vi "002 Data Forwarding Module.vi"(11 "Queue Ref In":T1={"UI"=refnum, "Message"=refnum, "Data"=refnum, "Caller"=refnum, "Name"="000 Common", "Data Path"=path "", "Class Path"=path "", "SubPanel"=refnum, "Project Name"="", "MNT"="", "Title"="", "Data Source"=refnum, "Queue List"={}, "VI"=refnum, "UE"=refnum}) -> ()   [LabVIEW 2020]
doc: "002 Data Forwarding Module.vi"
uses:
  Alin/QMH/000 Module Data Type.ctl
  Alin/QMH/Queue Message.ctl
  <vilib>/Utility/file.llb/Read Delimited Spreadsheet (string).vi
panel:
  in  "Forwarding Interval":u32=1000 caption="转发间隔(ms)" min=500 max=100000 step=1
  out "Name":string
  in  "Forward List":T2(array[cluster])
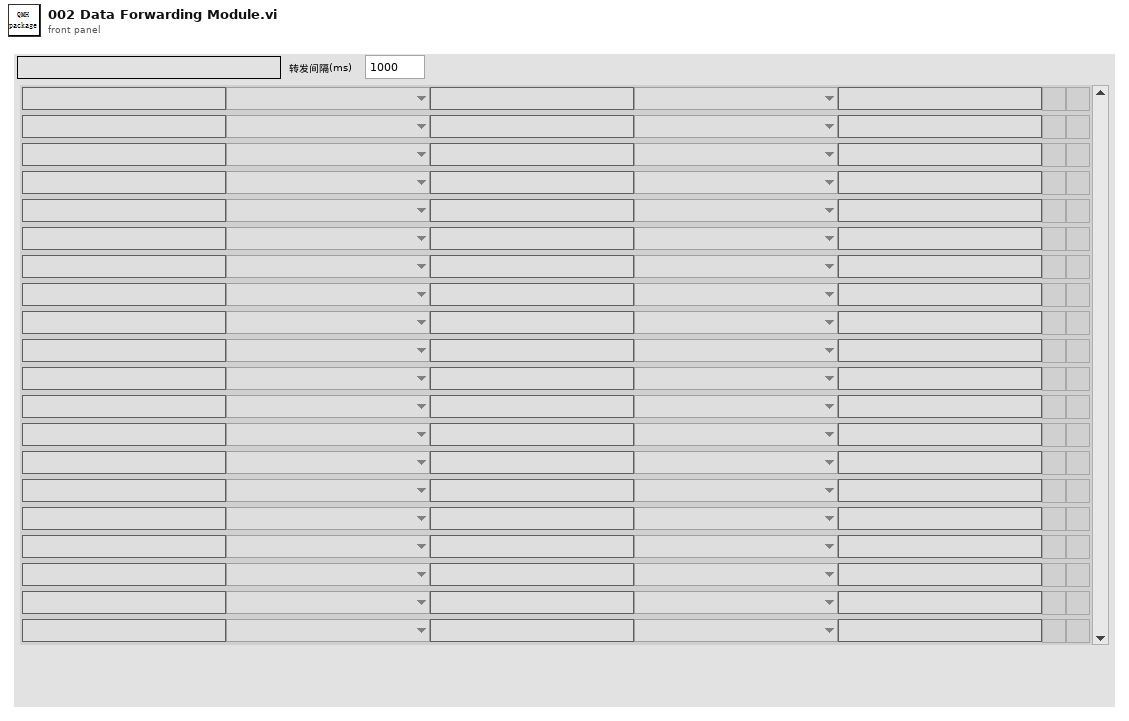
[diagram p1: front panel]
types:
  T1 = typedef "000 Module Data Type.ctl" = cluster{"UI":refnum<queue>, "Message":refnum<queue>, "Data":refnum<queue>, "Caller":refnum<queue>, "Name":string, "Data Path":path, "Class Path":path, "SubPanel":refnum<vi>, "Project Name":string, "MNT":string, "Title":string, "Data Source":refnum<queue>, "Queue List":map{string, refnum<queue>}, "VI":refnum<vi>, "UE":refnum<user-event>}
  T2 = cluster{"Name":string, "Sender":u16, "Send ID":string, "Receiver":u16, "Receive ID":string, "Edit":bool, "Delete":bool}[]
  T3 = cluster{"Queue":T1, "Delay":cluster{"Count Time(ms)":u32, "Delay Time(ms)":u32, "Next":string}, "Panel Name":string[], "Interval":u32, "Forward":map{string, cluster{"Name":string, "Sender":string, "SendID":string, "Receiver":string, "ReceiverID":string}}, "Group":map{string, map{string, cluster{"Name":string, "Sender":string, "SendID":string, "Receiver":string, "ReceiverID":string}}}, "Type":map{string, string}}
  T4 = map{string, cluster{"Name":string, "Sender":string, "SendID":string, "Receiver":string, "ReceiverID":string}}
  T5 = cluster{"all rows[0]":string, "all rows[1]":string, "all rows[2]":string, "all rows[3]":string, "all rows[4]":string}
  T6 = cluster{"Name":string, "Sender":string, "SendID":string, "Receiver":string, "ReceiverID":string}
  T7 = map{string, map{string, cluster{"Name":string, "Sender":string, "SendID":string, "Receiver":string, "ReceiverID":string}}}
  T8 = typedef "SDQ Data Type.ctl" = cluster{"CAN Length":string, "CAN Name":string, "CAN ID":string, "CAN Type":string, "Test Item":string, "Byte Order":string, "Instruction":string, "Control Type":string, "Group":string, "Offset":dbl, "Coefficient":dbl, "Write Enable":bool, "Lable Type":string, "Key?":string, "Set Value":string, "Upper":dbl, "Lower":dbl, "Unit":string, "Formula":string, "Test Item Type":string, "Length":i32, "Address":string, "Name":string, "Identifier":string, "Data Type":string, "Enumerate?":string, "Enumerate List":string, "Data":string, "Source":string}
  T9 = cluster{"Queue":T1, "Panel Name":string[], "Sender":refnum<vi>, "Receiver":refnum<vi>}
  T10 = typedef "eventvkey.ctl" = enum16{"ASCII", "Enter", "Return", "Shift", "Ctrl", "Alt", "Cmd", "Opt", "Caps", "NumLock", "Clear", "Break", "Up", "Down", "Left", "Right", "Insert", "Delete", "Home", "End", "PageUp", "PageDown", "Escape", "Help", "Pause", "ScrollLock", "F1", "F2", "F3", "F4", "F5", "F6", "F7", "F8", "F9", "F10", "F11", "F12", "F13", "F14", "F15", "F16", "F17", "F18", "F19", "F20", "F21", "F22", "F23", "F24", "Play", "VolumeUp", "VolumeDown", "Mute", "Two Byte Char"}
  T11 = cluster{"Shift":bool, "Ctrl":bool, "Alt":bool, "Cmd":bool, "Opt":bool}
  T12 = typedef "LVPoint32TypeDef.ctl" = cluster{"Horizontal":i32, "Vertical":i32}
  T13 = typedef "LVPositionTypeDef.ctl" = cluster{"Left":i32, "Top":i32}
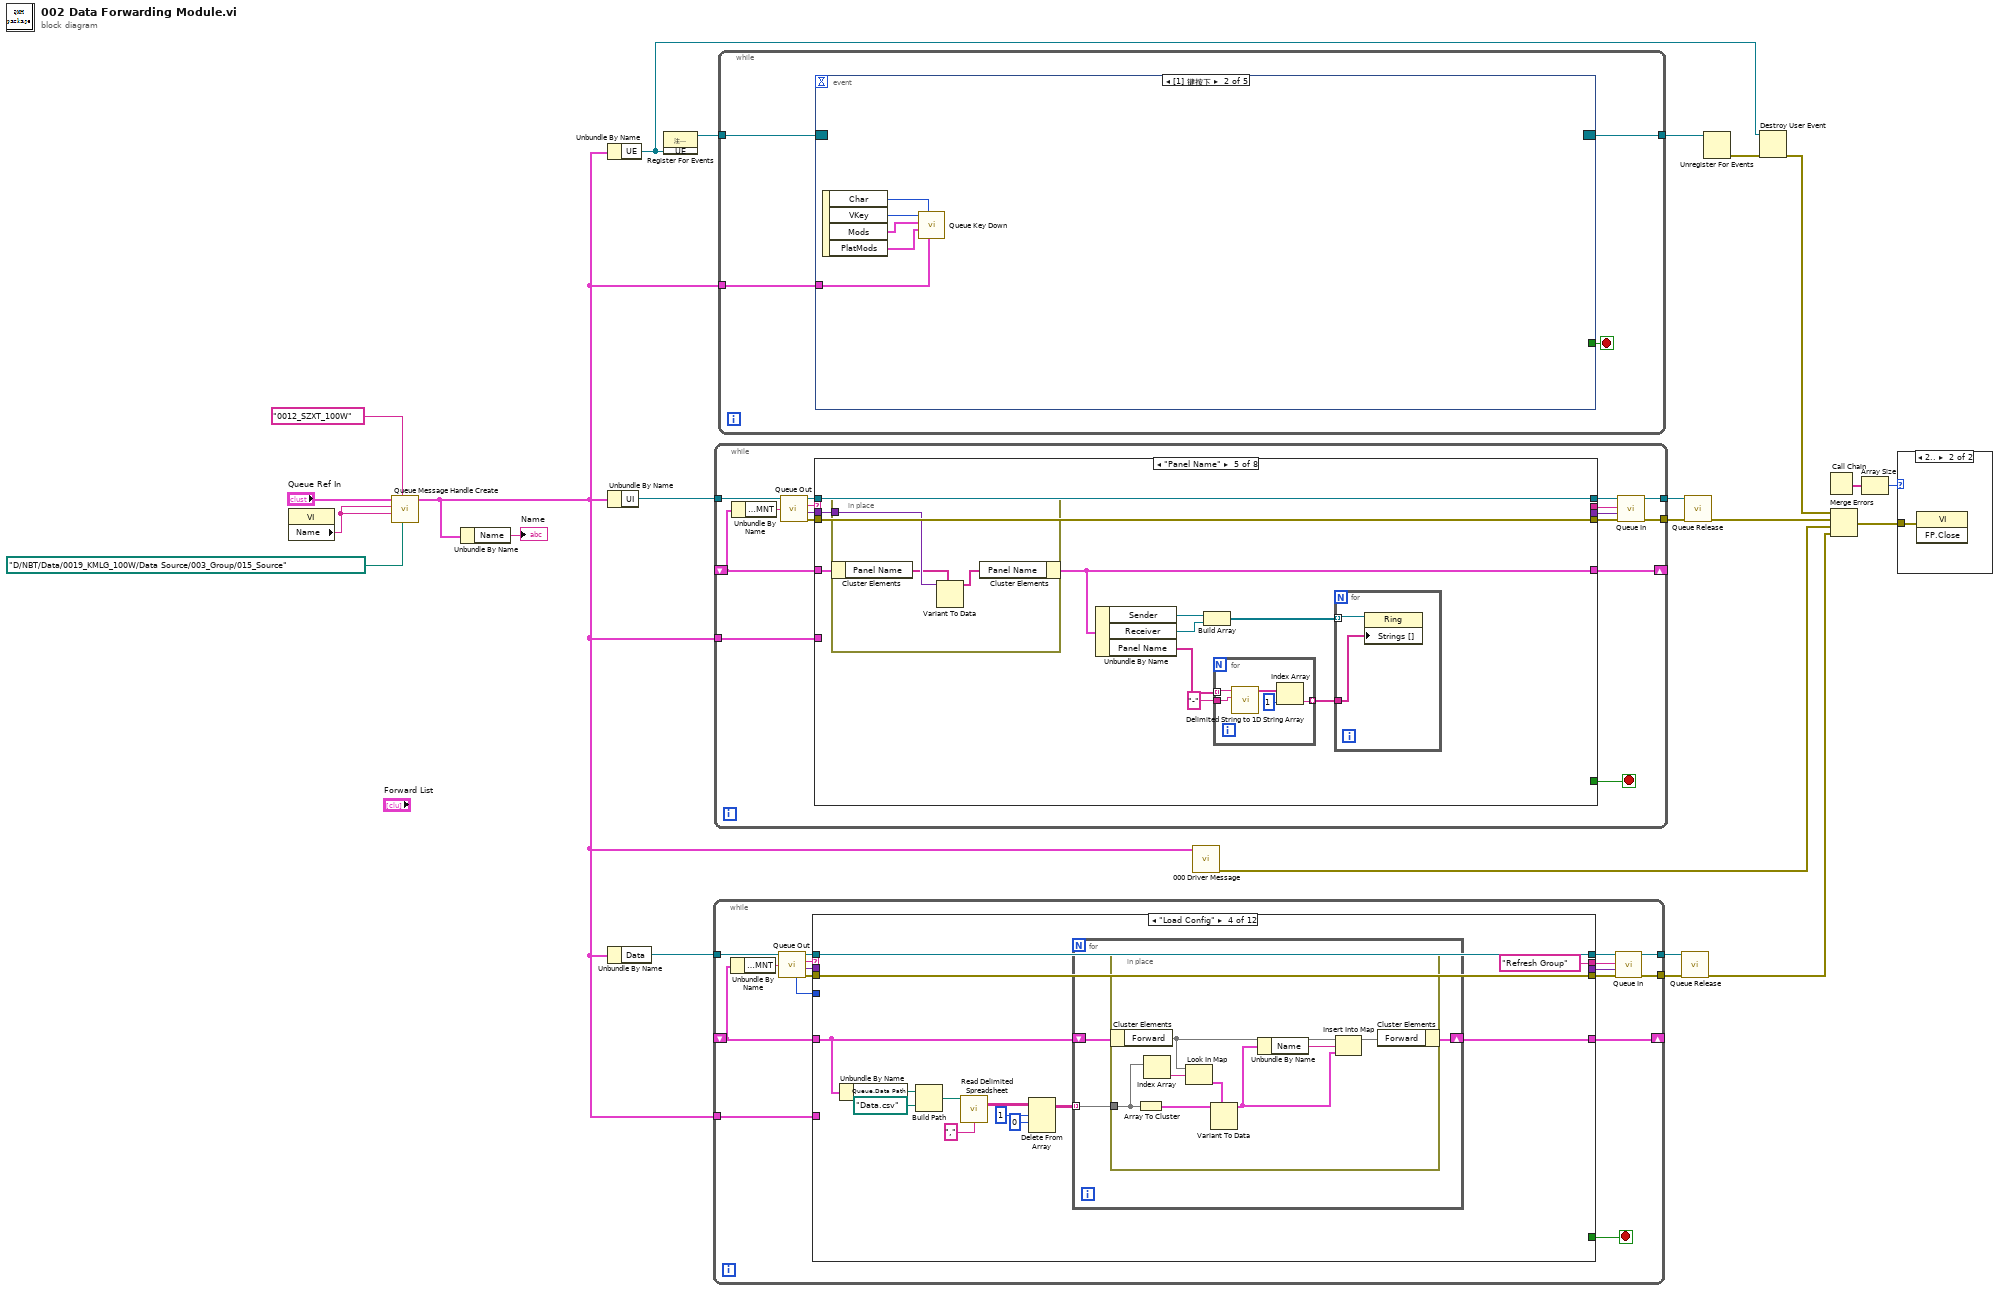
[diagram p0: block diagram]
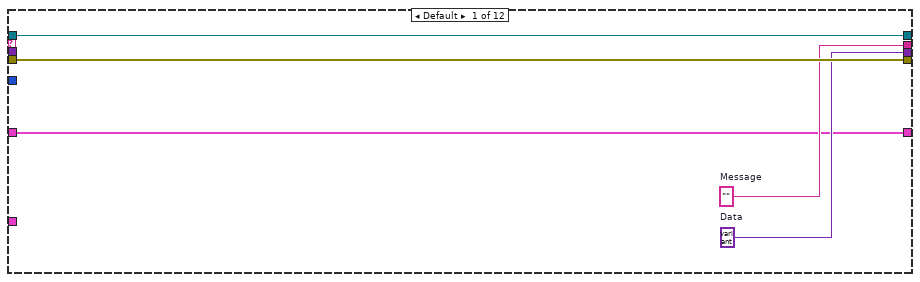
[diagram p2: hidden frame]
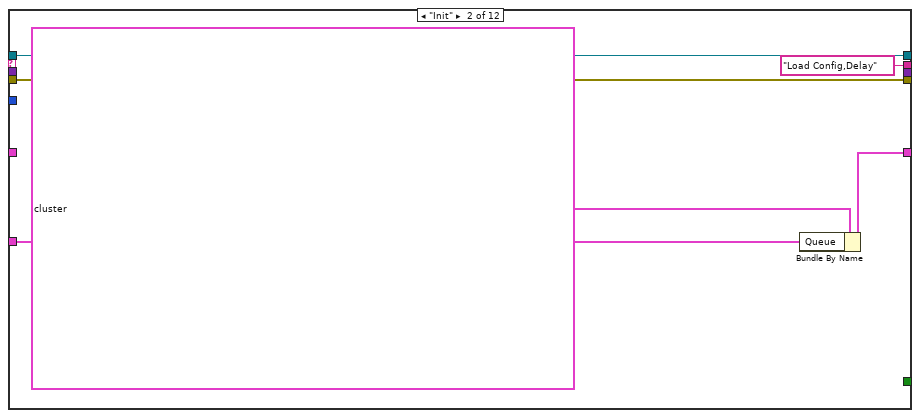
[diagram p3: hidden frame]
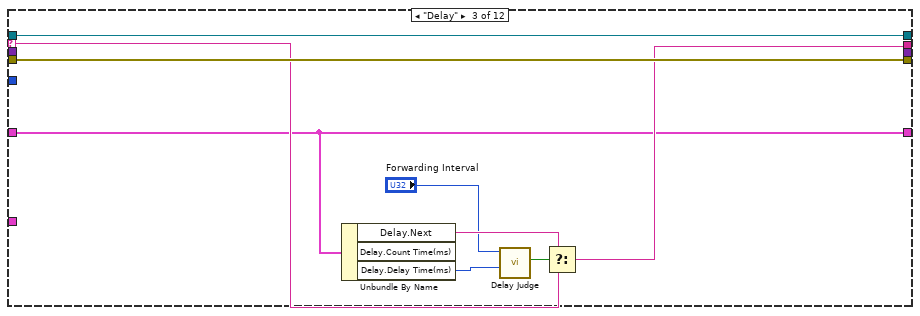
[diagram p4: hidden frame]
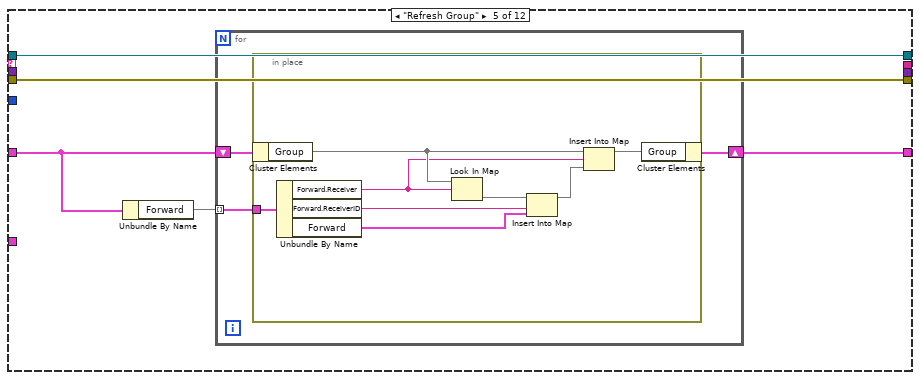
[diagram p5: hidden frame]
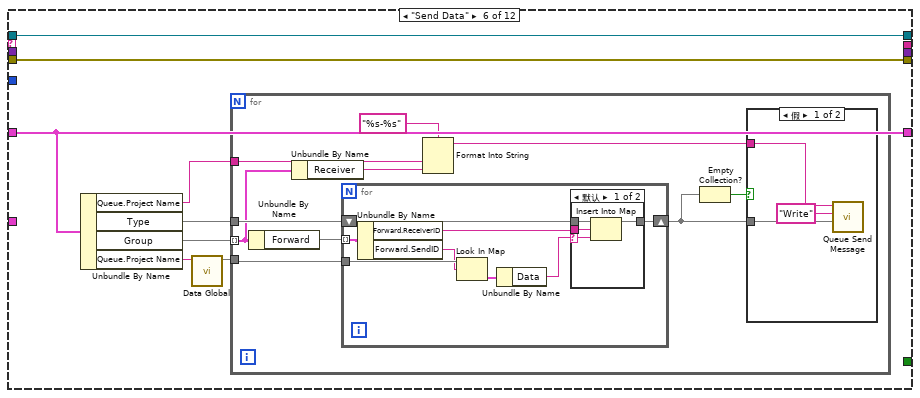
[diagram p6: hidden frame]
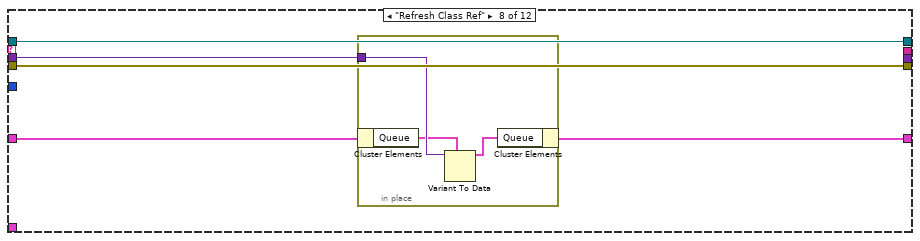
[diagram p10: hidden frame]
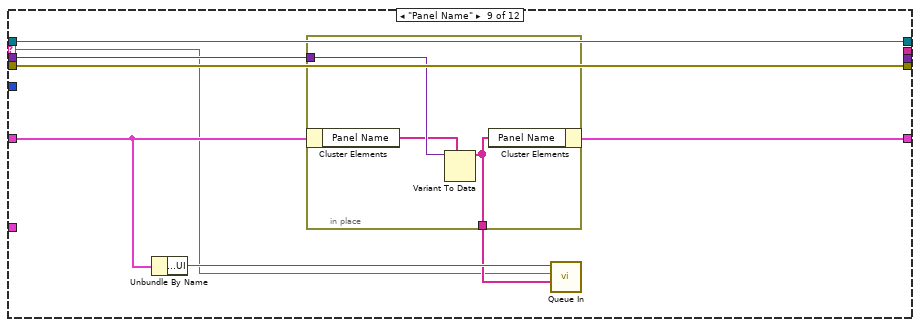
[diagram p11: hidden frame]
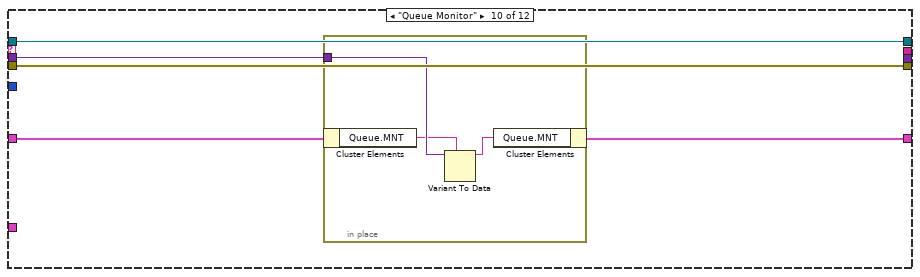
[diagram p12: hidden frame]
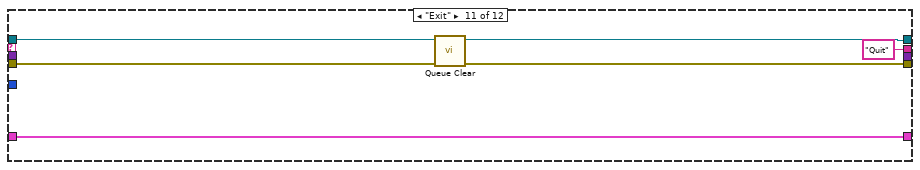
[diagram p13: hidden frame]
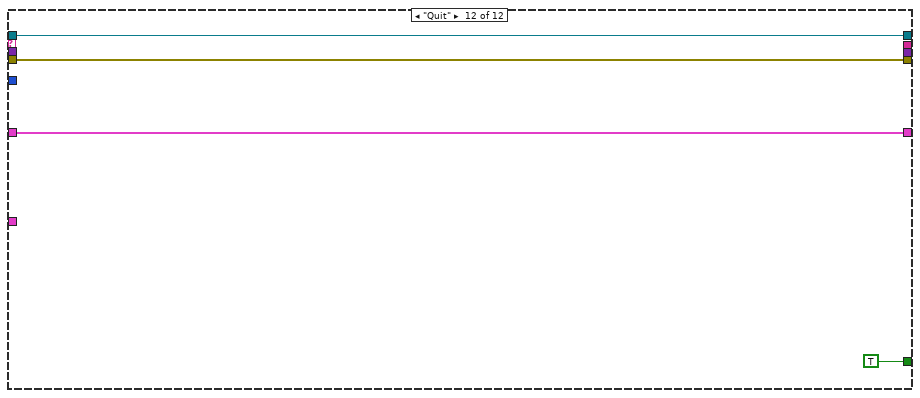
[diagram p14: hidden frame]
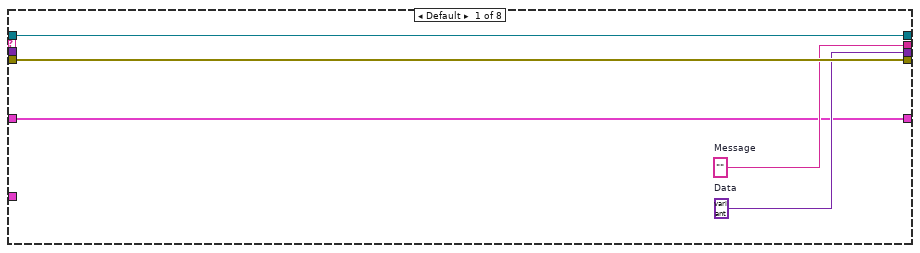
[diagram p16: hidden frame]
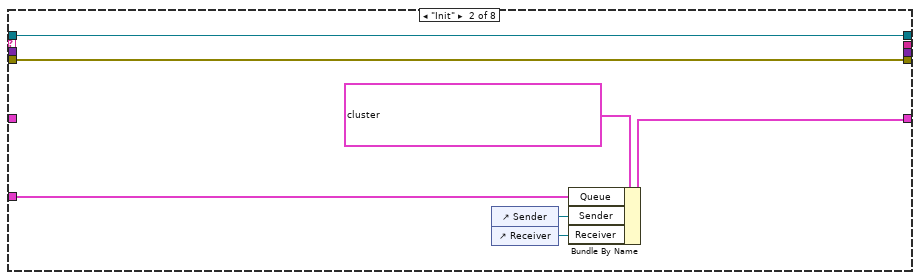
[diagram p17: hidden frame]
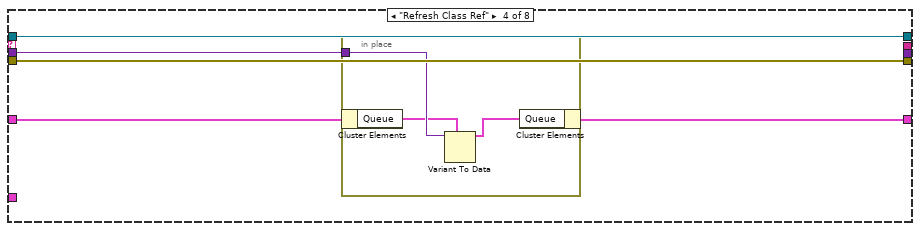
[diagram p19: hidden frame]
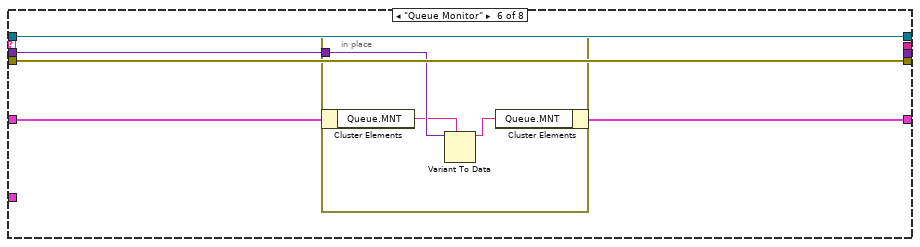
[diagram p20: hidden frame]
diagram:
  n1 = property class="VI"() -> ("Name"=w1:string)  [unwired: 2 in, 2 out]
  n2 = call "Queue Message Handle Create.vi"("Data Path"=path "D:/NBT/Data/0019_KMLG_100W/Data Source/003_Group/015_Source", "Project Name"="0012_SZXT_100W", "Name"=w1, "Title"=w1, "Queue Ref In"="Queue Ref In") -> ("Queue Ref Out"=w4:T1)  [unwired: 5 in, 1 out]
  n3 = Unbundle By Name(w4) -> ("Name"=→"Name":string)
  n4 = Unbundle By Name(w4) -> ("UE"=w7:refnum<user-event>)
  n5 = Unbundle By Name(w4) -> ("UI"=w18:refnum<queue>)
  n6 = Unbundle By Name(w4) -> ("Data"=w10:refnum<queue>)
  n7 = register-events(w7) -> (reference out=w23:refnum<event-registration>)  [unwired: 2 in, 1 out]
  n8 = while {
    tunnel: w10 -> [w36]
    tunnel: [w33] -> w12
    tunnel: [w32] -> w11
    shift-right: [w28] -> _
    shift-left: _ -> [w25]
    tunnel: w4 -> [w24]
    stop <- w40 stop-if-true
    n9 = Unbundle By Name(w25) -> ("Queue.MNT"=w26:string)
    n10 = call "Queue Out.vi"("Monitor"=w26, "Queue In"=w36) -> ("error out"=w39:errorcluster, "Data"=w37:variant, "Message"=w38:string, "Queue Out"=w35:refnum<queue>, "Queue NUmber"=w27:i32)  [unwired: 5 in]
    n11 = case shown="\"Load Config\"" w38 {
      selector: w38 -> [_ _ w54 _ _ _ _ _ w146 _ _ _]
      tunnel: w35 -> [w45 w51 w60 w73 w89 w108 w137 w142 w153 w161 w169 w173]
      tunnel: w39 -> [w44 w50 w59 w72 w88 w107 w136 w141 w152 w160 w167 w174]
      tunnel: [w45 w51 w60 w73 w89 w108 w137 w142 w153 w161 w168 w173] -> w34
      tunnel: [w44 w50 w59 w72 w88 w107 w136 w141 w152 w160 w166 w174] -> w31
      tunnel: [w43 "Load Config,Delay" ("Next") w55 "Refresh Group" ("Next") _ _ _ _ _ _ "Quit" _] -> w30
      tunnel: [_ _ _ _ _ _ _ _ _ _ _ TRUE] -> w40
      tunnel: [w42 _ _ _ _ _ _ _ _ _ _ _] -> w29
      tunnel: w37 -> [_ _ _ _ _ _ _ w138 w150 w157 _ _]
      tunnel: [w41 w47 w53 w63 w85 w106 w135 w139 w151 w158 w165 w171] -> w28
      tunnel: w25 -> [w41 _ w53 w64 w86 w106 w135 w140 w149 w159 w165 w171]
      tunnel: w27 -> [_ _ _ _ _ _ _ _ _ _ _ _]
      tunnel: w24 -> [_ w46 _ _ _ _ _ _ _ _ _ _]
      frame Default {
        w42 = variant  # Data
        w43 = ""  # Message
      }
      frame "Init" {
        n12 = Bundle By Name(cluster=T3 {"Queue"={"UI"=refnum, "Message"=refnum, "Data"=refnum, "Caller"=refnum, "Name"="000 Common", "Data Path"=path "", "Class Path"=path "", "SubPanel"=refnum, "Project Name"="", "MNT"="", "Title"="", "Data Source"=refnum, "Queue List"={}, "VI"=refnum, "UE"=refnum}, "Delay"={"Count Time(ms)"=1000, "Delay Time(ms)"=250, "Next"="Send Data,Delay"}, "Panel Name"=[], "Interval"=0, "Forward"={}, "Group"={}, "Type"={}}, "Queue"=w46) -> (w47:T3)
      }
      frame "Delay" {
        n13 = Unbundle By Name(w53) -> ("Delay.Next"=w58:string, "Delay.Delay Time(ms)"=w56:u32)  [unwired: 1 out]
        n14 = call "Delay Judge.vi"("Delay Time(ms)"=w56, "Count Time(ms)"="Forwarding Interval") -> ("Time Out?"=w57:bool)  [unwired: 5 in, 4 out]
        n15 = Select(t=w58, s=w57, f=w54) -> (s? t:f=w55:string)
      }
      frame "Load Config" {
        n16 = Unbundle By Name(w64) -> ("Queue.Data Path"=w71:path)
        n17 = Build Path(base path=w71, name or relative path=path "Data.csv" ("名称或相对路径")) -> (appended path=w69:path)
        n18 = call-poly <vilib>:"Read Delimited Spreadsheet.vi"("file path (dialog if empty)"=w69, "delimiter (\\t)"="," ("delimiter (\\t)")) -> ("all rows"=w67:string[][])  [unwired: 8 in, 5 out]
        n19 = Delete From Array(array=w67, length=1 ("长度"), index (row)=0 ("索引 (行)")) -> (array with subset deleted=w62:string[][])  [unwired: 1 in, 1 out]
        n20 = for {
          shift-right: [w75] -> w63
          shift-left: w64 -> [w76]
          tunnel: w62 -> [w74] mode=indexing
          n21 = in-place {
            in-place-border: w74 -> [w83]
            n22 = in-place-cluster #1(w76) -> ("Forward"=w81:T4)
            n23 = Array To Cluster(array=w83) -> (cluster=w84:T5)
            n24 = Index Array(array=w83) -> (element=w82:string)  [unwired: 1 in]
            n25 = Look In Map(map=w81, key=w82) -> (value=w78:T6)  [unwired: 1 in, 1 out]
            n26 = Variant To Data(type=w78, Variant=w84) -> (data=w77:T6)  [unwired: 1 in, 1 out]
            n27 = Unbundle By Name(w77) -> ("Name"=w79:string)
            n28 = Insert Into Map(map in=w81, key=w79, value=w77) -> (map out=w80:T4)  [unwired: 2 out]
            n29 = in-place-cluster #1("Forward"=w80) -> (w75:T3)
          }
        }
      }
      frame "Refresh Group" {
        n30 = Unbundle By Name(w86) -> ("Forward"=w87:T4)
        n31 = for {
          tunnel: w87 -> [w90] mode=indexing
          shift-right: [w91] -> w85
          shift-left: w86 -> [w92]
          n32 = in-place {
            in-place-border: w90 -> [w100]
            n33 = in-place-cluster #2(w92) -> ("Group"=w98:T7)
            n34 = Unbundle By Name(w100) -> ("Forward.Receiver"=w95:string, "Forward.ReceiverID"=w94:string, "Forward"=w93:T6)
            n35 = Look In Map(map=w98, key=w95) -> (value=w99:T4)  [unwired: 1 in, 1 out]
            n36 = Insert Into Map(map in=w99, key=w94, value=w93) -> (map out=w96:T4)  [unwired: 2 out]
            n37 = Insert Into Map(map in=w98, key=w95, value=w96) -> (map out=w97:T7)  [unwired: 2 out]
            n38 = in-place-cluster #2("Group"=w97) -> (w91:T3)
          }
        }
      }
      frame "Send Data" {
        n39 = Unbundle By Name(w106) -> ("Queue.Project Name"=w101:string, "Type"=w102:map{string, string}, "Group"=w104:T7, "Queue.Project Name"=w105:string)
        n40 = call "Data Global.vi"("Name"=w105) -> ("Data Out"=w103:map{string, T8})  [unwired: 7 in, 3 out]
        n41 = for {
          tunnel: w104 -> [w113] mode=indexing
          tunnel: w103 -> [w118]
          tunnel: w102 -> [w116]
          tunnel: w101 -> [w114]
          n42 = Unbundle By Name(w113) -> ("Forward"=w117:T4)
          n43 = Unbundle By Name(w113) -> ("Receiver"=w112:string)
          n44 = for {
            tunnel: w118 -> [w129]
            tunnel: w117 -> [w125] mode=indexing
            shift-right: [w126] -> w110
            shift-left: w116 -> [w127]
            n45 = Unbundle By Name(w125) -> ("Forward.ReceiverID"=w122:string, "Forward.SendID"=w124:string)
            n46 = Look In Map(map=w129, key=w124) -> (value=w128:T8)  [unwired: 1 in, 1 out]
            n47 = Unbundle By Name(w128) -> ("Data"=w123:string)
            n48 = case shown="默认" w123 {
              selector: w123 -> [w130 _]
              tunnel: w127 -> [w133 w134]
              tunnel: [w132 w134] -> w126
              tunnel: w122 -> [w131 _]
              frame Default {
                n49 = Insert Into Map(map in=w133, key=w131, value=w130) -> (map out=w132:map{string, string})  [unwired: 2 out]
              }
              frame "" {
              }
            }
          }
          n50 = Format Into String(format string="%s-%s" ("格式字符串"), w114, w112) -> (resulting string=w111:string)  [unwired: 2 in, 1 out]
          n51 = Empty Collection?(1:w110) -> (0:w109:bool)
          n52 = case shown="假" w109 {
            tunnel: w111 -> [w120 _]
            tunnel: w110 -> [w119 _]
            frame False {
              n53 = call "Queue Send Message.vi"("Data"=w119, "Message"="Write", "Queue Name"=w120) -> ()  [unwired: 6 in, 3 out]
            }
            frame True {
            }
          }
        }
      }
      frame "====System====" {
      }
      frame "Refresh Class Ref" {
        n54 = in-place {
          in-place-border: w138 -> [w145]
          n55 = in-place-cluster #3(w140) -> ("Queue"=w144:T1)
          n56 = Variant To Data(type=w144, Variant=w145) -> (data=w143:T1)  [unwired: 1 in, 1 out]
          n57 = in-place-cluster #3("Queue"=w143) -> (w139:T3)
        }
      }
      frame "Panel Name" {
        n58 = Unbundle By Name(w149) -> ("Queue.UI"=w148:refnum<queue>)
        n59 = in-place {
          in-place-border: w150 -> [w156]
          in-place-border: [w154] -> w147
          n60 = in-place-cluster #4(w149) -> ("Panel Name"=w155:string[])
          n61 = Variant To Data(type=w155, Variant=w156) -> (data=w154:string[])  [unwired: 1 in, 1 out]
          n62 = in-place-cluster #4("Panel Name"=w154) -> (w151:T3)
        }
        n63 = call "Queue In.vi"("Data"=w147, "Message"=w146, "Queue In"=w148) -> ()  [unwired: 7 in, 2 out]
      }
      frame "Queue Monitor" {
        n64 = in-place {
          in-place-border: w157 -> [w164]
          n65 = in-place-cluster #5(w159) -> ("Queue.MNT"=w163:string)
          n66 = Variant To Data(type=w163, Variant=w164) -> (data=w162:string)  [unwired: 1 in, 1 out]
          n67 = in-place-cluster #5("Queue.MNT"=w162) -> (w158:T3)
        }
      }
      frame "Exit" {
        n68 = call "Queue Clear.vi"("error in (no error)"=w167, "Queue In"=w169) -> ("error out"=w166:errorcluster, "Queue Out"=w168:refnum<queue>)  [unwired: 8 in]
      }
      frame "Quit" {
      }
    }
    n69 = call "Queue In.vi"("error in (no error)"=w31, "Data"=w29, "Message"=w30, "Queue In"=w34) -> ("error out"=w32:errorcluster, "Queue Out"=w33:refnum<queue>)  [unwired: 6 in]
  }
  n70 = while {
    tunnel: w18 -> [w186]
    tunnel: [w183] -> w20
    tunnel: [w182] -> w19
    shift-right: [w178] -> _
    shift-left: _ -> [w177]
    tunnel: w4 -> [w175]
    stop <- w190 stop-if-true
    n71 = Unbundle By Name(w177) -> ("Queue.MNT"=w176:string)
    n72 = call "Queue Out.vi"("Monitor"=w176, "Queue In"=w186) -> ("error out"=w189:errorcluster, "Data"=w187:variant, "Message"=w188:string, "Queue Out"=w185:refnum<queue>)  [unwired: 5 in, 1 out]
    n73 = case shown="\"Panel Name\"" w188 {
      selector: w188 -> [_ _ _ _ _ _ w245 _]
      tunnel: w185 -> [w195 w202 w205 w210 w224 w239 w252 w258]
      tunnel: w189 -> [w194 w201 w204 w209 w223 w238 w250 w259]
      tunnel: [w195 w202 w205 w210 w224 w239 w251 w258] -> w184
      tunnel: [w194 w201 w204 w209 w223 w238 w249 w259] -> w181
      tunnel: [w193 _ _ _ _ _ "Quit" _] -> w180
      tunnel: [_ _ _ _ _ _ _ TRUE] -> w190
      tunnel: [w192 _ _ _ _ _ _ _] -> w179
      tunnel: w187 -> [_ _ _ w206 w221 w235 _ _]
      tunnel: [w191 w199 w203 w207 w220 w236 w244 w256] -> w178
      tunnel: w177 -> [w191 _ w203 w208 w222 w237 w244 w256]
      tunnel: w175 -> [_ w198 _ _ _ _ _ _]
      frame Default {
        w192 = variant  # Data
        w193 = ""  # Message
      }
      frame "Init" {
        n74 = control-ref of="Sender"() -> (w197:refnum<vi>)
        n75 = control-ref of="Receiver"() -> (w196:refnum<vi>)
        n76 = Bundle By Name(cluster=T9 {"Queue"={"UI"=refnum, "Message"=refnum, "Data"=refnum, "Caller"=refnum, "Name"="000 Common", "Data Path"=path "", "Class Path"=path "", "SubPanel"=refnum, "Project Name"="", "MNT"="", "Title"="", "Data Source"=refnum, "Queue List"={}, "VI"=refnum, "UE"=refnum}, "Panel Name"=[], "Sender"=refnum, "Receiver"=refnum}, "Queue"=w198, "Sender"=w197, "Receiver"=w196) -> (w199:T9)
      }
      frame "====System====" {
      }
      frame "Refresh Class Ref" {
        n77 = in-place {
          in-place-border: w206 -> [w213]
          n78 = in-place-cluster #6(w208) -> ("Queue"=w212:T1)
          n79 = Variant To Data(type=w212, Variant=w213) -> (data=w211:T1)  [unwired: 1 in, 1 out]
          n80 = in-place-cluster #6("Queue"=w211) -> (w207:T9)
        }
      }
      frame "Panel Name" {
        n81 = in-place {
          in-place-border: w221 -> [w234]
          n82 = in-place-cluster #7(w222) -> ("Panel Name"=w233:string[])
          n83 = Variant To Data(type=w233, Variant=w234) -> (data=w232:string[])  [unwired: 1 in, 1 out]
          n84 = in-place-cluster #7("Panel Name"=w232) -> (w220:T9)
        }
        n85 = Unbundle By Name(w220) -> ("Sender"=w219:refnum<vi>, "Receiver"=w218:refnum<vi>, "Panel Name"=w216:string[])
        n86 = Build Array(w219, w218) -> (w217:refnum<vi>[])
        n87 = for {
          tunnel: w216 -> [w229] mode=indexing
          tunnel: "-" ("delimiter") -> [w228]
          tunnel: [w226] -> w214 mode=indexing
          n88 = call <vilib>:"Delimited String to 1D String Array.vi"("delimiter"=w228, "delimited string"=w229) -> ("string array"=w227:string[])  [unwired: 9 in]
          n89 = Index Array(array=w227, index=1 ("索引")) -> (element=w226:string)
        }
        n90 = for {
          tunnel: w217 -> [w231] mode=indexing
          tunnel: w214 -> [w230]
          n91 = property class="Ring"(reference=w231, "Strings []"=w230) -> ()  [unwired: 1 in, 2 out]
        }
      }
      frame "Queue Monitor" {
        n92 = in-place {
          in-place-border: w235 -> [w242]
          n93 = in-place-cluster #8(w237) -> ("Queue.MNT"=w241:string)
          n94 = Variant To Data(type=w241, Variant=w242) -> (data=w240:string)  [unwired: 1 in, 1 out]
          n95 = in-place-cluster #8("Queue.MNT"=w240) -> (w236:T9)
        }
      }
      frame "Exit" {
        n96 = Unbundle By Name(w244) -> ("Queue.Message"=w248:refnum<queue>, "Queue.Data"=w247:refnum<queue>, "Queue.UE"=w243:refnum<user-event>)
        n97 = Build Array(w248, w247) -> (w246:refnum<queue>[])
        n98 = Generate User Event(user event=w243, event data cluster=w245) -> ()  [unwired: 2 in, 2 out]
        n99 = for {
          tunnel: w246 -> [w255] mode=indexing
          tunnel: w245 -> [w254]
          n100 = call "Queue In.vi"("Message"=w254, "Queue In"=w255) -> ()  [unwired: 8 in, 2 out]
        }
        n101 = call "Queue Clear.vi"("error in (no error)"=w250, "Queue In"=w252) -> ("error out"=w249:errorcluster, "Queue Out"=w251:refnum<queue>)  [unwired: 8 in]
      }
      frame "Quit" {
      }
    }
    n102 = call "Queue In.vi"("error in (no error)"=w181, "Data"=w179, "Message"=w180, "Queue In"=w184) -> ("error out"=w182:errorcluster, "Queue Out"=w183:refnum<queue>)  [unwired: 6 in]
  }
  n103 = while {
    tunnel: w23 -> [w263]
    tunnel: [w261] -> w22
    tunnel: w4 -> [w260]
    stop <- w262 stop-if-true
    n104 = event shown="[1] 键按下" {
      selector: w263 -> [_ _ _ _ _]
      dyn-events: [_ _ _ _ _] -> w261
      timeout: _ -> [_ _ _ _ _]
      tunnel: [_ _ w269 _ _] -> w262
      tunnel: w260 -> [_ w267 _ _ w279]
      event Timeout {
        n105 = event-data() -> ()  [unwired: 1 in, 1 out]
      }
      event Key Down {
        n106 = event-data() -> ("Char"=w268:i16, "VKey"=w266:T10, "Mods"=w265:cluster{"Num Pad":bool, "Menu Key":bool}, "PlatMods"=w264:T11)  [unwired: 1 in]
        n107 = call "Queue Key Down.vi"("Queue Ref Out"=w267, "C"=w268, "Platform Key"=w264, "Group Key"=w265, "V Key"=w266) -> ()  [unwired: 6 in, 1 out]
      }
      event User Event {
        n108 = event-data() -> ("Message"=w271:string)  [unwired: 1 in]
        n109 = Equal?(x=w271, y="Exit") -> (x = y?=w269:bool)
      }
      event "Forward List": Mouse Down {
        n110 = event-data() -> ("Coords"=w276:T12, "CtlRef"=w273:refnum<vi>)  [unwired: 1 in]
        n111 = property class="Arr"(reference=w273) -> ("Position"=w275:T13, "Array Element.Height"=w272:u32)  [unwired: 1 in, 2 out]
        n112 = Subtract(x=w276, y=w275) -> (x-y=w274:T12)
        n113 = Divide(x=w274, y=w272) -> ()  [unwired: 1 out]
      }
      event Panel Close? {
        n114 = event-data() -> ()  [unwired: 1 in, 1 out]
        n115 = Call Chain() -> (call chain=w281:string[])
        n116 = Array Size(array=w281) -> (size(s)=w280:i32)
        n117 = case shown="2, 默认" w280 {
          tunnel: w279 -> [w285 w288]
          tunnel: [w284 w287] -> w278
          tunnel: ["Panel Hidden" ("Message") "Exit Prepare" ("Message")] -> w277
          frame 2, Default {
            n118 = Unbundle By Name(w285) -> ("Message"=w284:refnum<queue>)
          }
          frame 1 {
            n119 = Unbundle By Name(w288) -> ("Message"=w287:refnum<queue>)
          }
        }
        n120 = call "Queue In.vi"("Message"=w277, "Queue In"=w278) -> ()  [unwired: 8 in, 2 out]
        n121 = event-data("Discard?"=TRUE ("放弃？")) -> ()  [unwired: 1 in, 1 out]
      }
    }
  }
  n122 = call "000 Driver Message.vi"("Queue In"=w4) -> ("error out"=w8:errorcluster)  [unwired: 8 in, 2 out]
  n123 = call "Queue Release.vi"("error in (no error)"=w11, "Queue In"=w12) -> ("error out"=w9:errorcluster)  [unwired: 9 in]
  n124 = call "Queue Release.vi"("error in (no error)"=w19, "Queue In"=w20) -> ("error out"=w16:errorcluster)  [unwired: 9 in]
  n125 = Unregister For Events(event registration refnum=w22) -> (error out=w21:errorcluster)  [unwired: 1 in]
  n126 = Destroy User Event(user event=w7, error in=w21) -> (error out=w17:errorcluster)
  n127 = Call Chain() -> (call chain=w14:string[])
  n128 = Merge Errors(w17, w16, w8, w9) -> (w15:errorcluster)
  n129 = Array Size(array=w14) -> (size(s)=w13:i32)
  n130 = case shown="2.." w13 {
    tunnel: w15 -> [_ w289]
    frame 0, Default {
    }
    frame 2.. {
      n131 = invoke class="VI" method="FP.Close"(error in=w289) -> ()  [unwired: 2 in, 3 out]
    }
  }
